vi "read_from_stream_rocket_data.vi"() -> ()   [LabVIEW 2018]
uses:
  <vilib>/Utility/sysdir.llb/System Directory Type.ctl
  <resource>/objmgr/ni.dex.rc
panel:
  in  "name or relative path":string
  out "Connected to MyRio":bool
  out "error out":errorcluster
  in  "Start Saving Data":bool
  in  "stop":bool
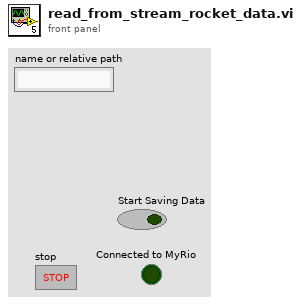
[diagram p1: front panel]
types:
  T1 = enum16{"open", "replace", "create", "open or create", "replace or create", "replace or create with confirmation"}
  T2 = typedef "System Directory Type.ctl" = i32
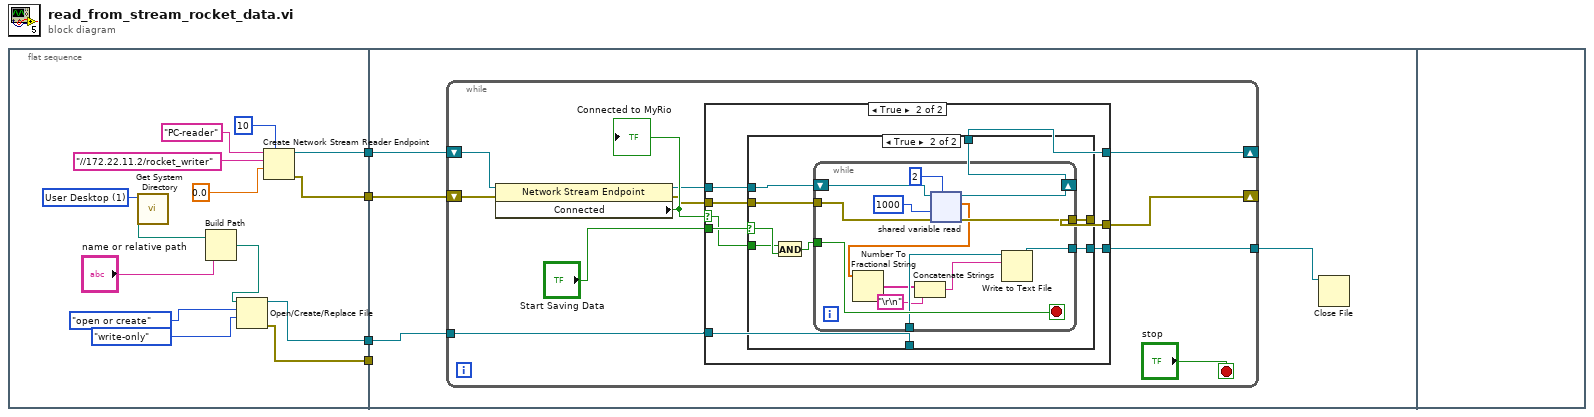
[diagram p0: block diagram]
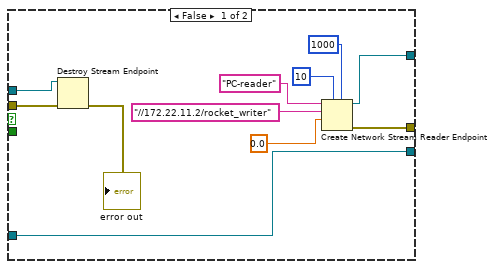
[diagram p2: hidden frame]
diagram:
  n1 = flat-sequence {
    tunnel: [w16] -> w4
    tunnel: [w11] -> w3
    tunnel: [w10] -> w2
    tunnel: [w9] -> w1
    tunnel: w4 -> [w22]
    tunnel: w3 -> [w20]
    tunnel: w2 -> [_]
    tunnel: w1 -> [w21]
    frame #0 {
      w5 = T2 1 items=["User Home"=0, "User Desktop"=1, "User Documents"=2, "User Application Data"=3, "User Preferences"=4, "User Temporary"=5, "Public Documents"=6, "Public Application Data"=7, "Public Preferences"=8, "Public Cache"=13, "System Core Libraries"=9, "System Installed Libraries"=10, "Application Files"=11, "Boot Volume Root"=12] ("system directory type")
      n2 = call <vilib>:"Get System Directory.vi"("system directory type"=w5) -> ("system directory"=w6:path)  [unwired: 10 in]
      n3 = Build Path(base path=w6, name or relative path="name or relative path") -> (appended path=w7:path)
      n4 = Open/Create/Replace File(file path (use dialog)=w7, operation (0:open)=T1."open or create", access (0:read/write)=enum16{"read/write", "read-only", "write-only"}."write-only") -> (refnum out=w11:refnum<file>, error out=w10:errorcluster)  [unwired: 3 in, 1 out]
      n5 = Create Network Stream Reader Endpoint(7:10 ("reader buffer size"), 9:0.0, 10:"//172.22.11.2/rocket_writer" ("writer url"), 11:"PC-reader" ("reader name")) -> (0:w9:errorcluster, 3:w16:refnum<k21>)  [unwired: 3 in]
    }
    frame #1 {
      n6 = while {
        shift-right: [w29] -> _
        shift-left: w22 -> [w32]
        shift-right: [w26] -> _
        shift-left: w21 -> [w28]
        tunnel: w20 -> [w25]
        tunnel: [w24] -> w19
        stop <- "stop" stop-if-true
        n7 = property class="Network Stream Endpoint"(reference=w32, error in=w28) -> (reference out=w30:refnum<k21>, error out=w27:errorcluster, "Connected"=w31:bool)
        "Connected to MyRio" <- w31
        n8 = case shown="True" w31 {
          selector: w31 -> [_ w49]
          tunnel: w30 -> [w36 w52]
          tunnel: "Start Saving Data" -> [_ w51]
          tunnel: [w40 w50] -> w29
          tunnel: w27 -> [w39 w48]
          tunnel: [w37 w47] -> w26
          tunnel: w25 -> [w34 w46]
          tunnel: [w34 w45] -> w24
          frame False {
            n9 = Destroy Stream Endpoint(8:w39, 11:w36) -> (0:→"error out":errorcluster)
            n10 = Create Network Stream Reader Endpoint(5:1000 ("timeout in ms (-1)"), 7:10 ("reader buffer size"), 9:0.0, 10:"//172.22.11.2/rocket_writer" ("writer url"), 11:"PC-reader" ("reader name")) -> (0:w37:errorcluster, 3:w40:refnum<k21>)  [unwired: 2 in]
          }
          frame True {
            n11 = case shown="True" w51 {
              selector: w51 -> [_ w62]
              tunnel: w52 -> [w55 w64]
              tunnel: [w55 w63] -> w50
              tunnel: w49 -> [_ w61]
              tunnel: w48 -> [w54 w59]
              tunnel: [w54 w58] -> w47
              tunnel: w46 -> [w53 w57]
              tunnel: [w53 w56] -> w45
              frame False {
              }
              frame True {
                n12 = And(x=w61, y=w62) -> (x .and. y?=w60:bool)
                n13 = while {
                  shift-right: [w75] -> w63
                  shift-left: w64 -> [w77]
                  tunnel: w60 -> [w74]
                  tunnel: w59 -> [w73]
                  tunnel: [w72] -> w58
                  tunnel: w57 -> [w71]
                  tunnel: [w69] -> w56
                  stop <- w74 stop-if-true
                  n14 = shared-variable-read(w77, w73, 1000 ("timeout ms (-1)"), 2 ("# elements")) -> (w75:refnum<k21>, w72:errorcluster, w70:dbl[])  [unwired: 1 out]
                  n15 = Number To Fractional String(number=w70) -> (F-format string=w68:string[])  [unwired: 3 in]
                  n16 = Concatenate Strings(w68, "\r\n") -> (w67:string)
                  n17 = Write to Text File(file (use dialog)=w71, text=w67) -> (refnum out=w69:refnum<file>)  [unwired: 2 in, 2 out]
                }
              }
            }
          }
        }
      }
      n18 = Close File(refnum=w19) -> ()  [unwired: 1 in, 2 out]
    }
    frame #2 {
    }
  }
